vi "Media_VF.2.vi"(1 "Nota da VC":dbl, 2 "Notas da VE":dbl[](array[numeric])) -> (0 "Nota da VF":dbl)   [LabVIEW 2018]
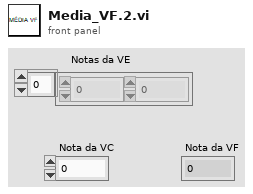
[diagram p1: front panel]
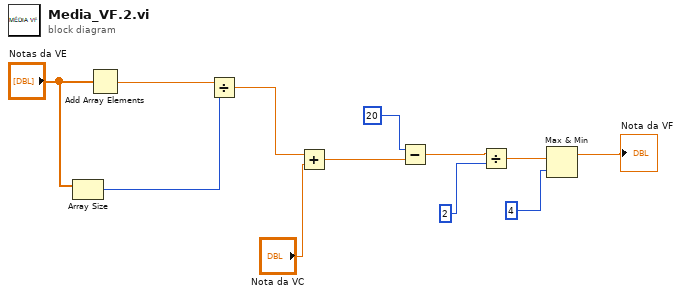
[diagram p0: block diagram]
diagram:
  n1 = Array Size(array="Notas da VE") -> (size(s)=w11:i32)
  n2 = Add Array Elements(numeric array="Notas da VE") -> (sum=w12:dbl)
  n3 = Divide(x=w12, y=w11) -> (x/y=w9:dbl)
  n4 = Add(x=w9, y="Nota da VC") -> (x+y=w7:dbl)
  n5 = Subtract(x=20, y=w7) -> (x-y=w5:dbl)
  n6 = Divide(x=w5, y=2) -> (x/y=w3:dbl)
  n7 = Max & Min(x=w3, y=4) -> (max(x,y)=→"Nota da VF":dbl)  [unwired: 1 out]
